vi "PCE_TCP_CMD.vi"(0 "CID IN":refnum<k5>, 7 "Timeout":u32=25 min=10 step=1, 11 "Error IN":errorcluster) -> (4 "CID OUT":refnum<k5>, 6 "FIFOelt":cluster{string, "data out":string, string}, 10 "Cmd?":bool, 15 "Error OUT":errorcluster)   [LabVIEW 2011]
panel:
  out "ExecTime":u32
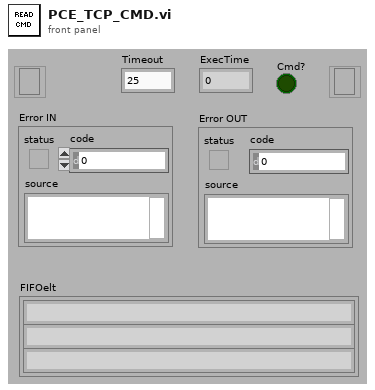
[diagram p1: front panel]
types:
  T1 = enum16{"Standard", "Buffered", "CRLF", "Immediate"}
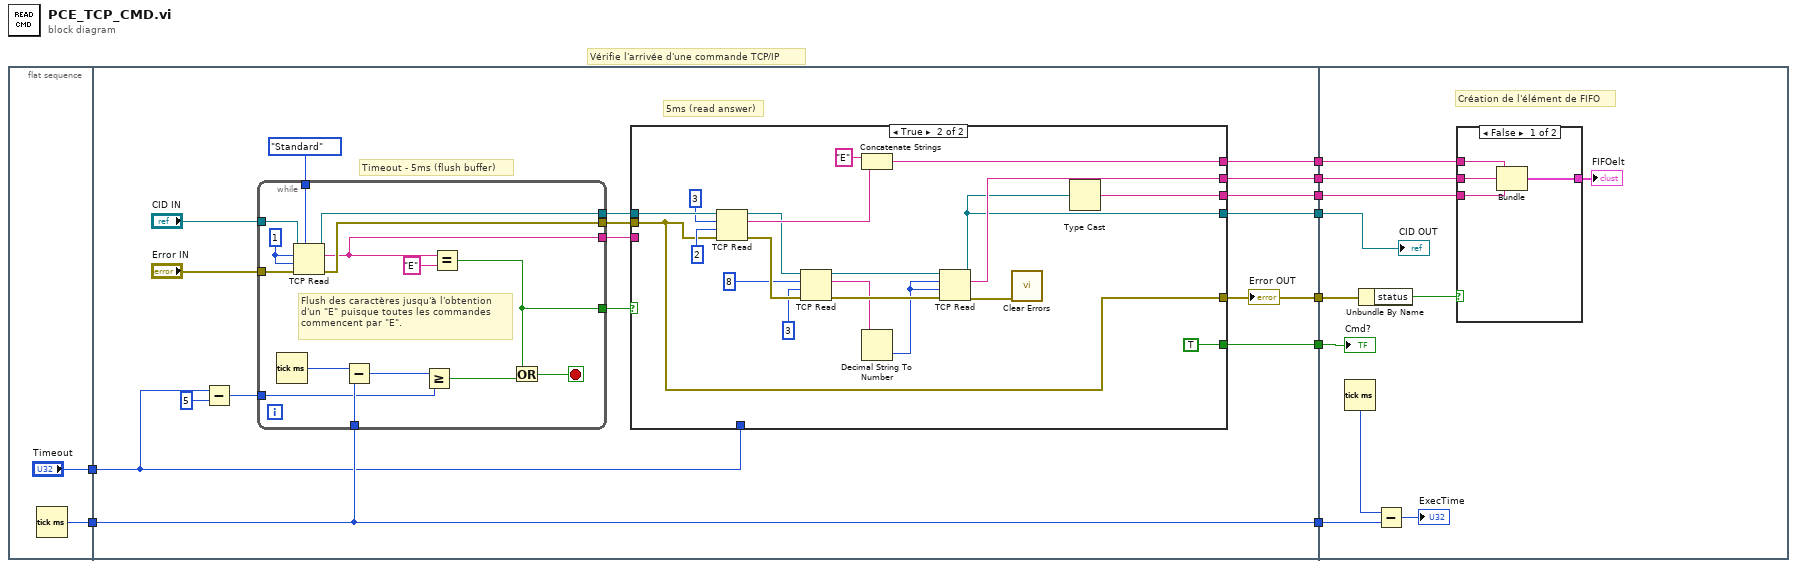
[diagram p0: block diagram]
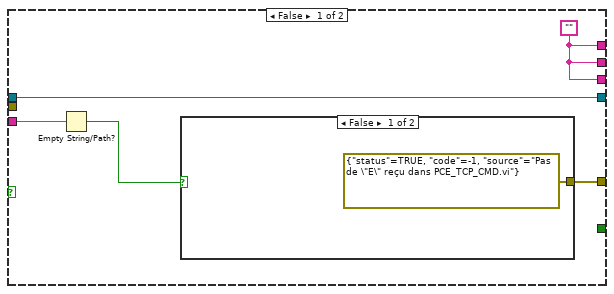
[diagram p2: hidden frame]
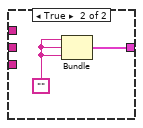
[diagram p4: hidden frame]
diagram:
  # "Vérifie l'arrivée d'une commande TCP/IP"
  n1 = flat-sequence {
    tunnel: [w11] -> w9
    tunnel: ["Timeout"] -> w7
    tunnel: w9 -> [w28]
    tunnel: [w28] -> w8
    tunnel: w7 -> [w20]
    tunnel: [w19] -> w6
    tunnel: [w18] -> w5
    tunnel: [w17] -> w4
    tunnel: [w16] -> w3
    tunnel: [w15] -> w2
    tunnel: [w12] -> w1
    tunnel: w8 -> [w80]
    tunnel: w6 -> [w71]
    tunnel: w5 -> [w77]
    tunnel: w4 -> [w75]
    tunnel: w3 -> [w74]
    tunnel: w2 -> [w73]
    tunnel: w1 -> [w70]
    frame #0 {
      n2 = Tick Count (ms)() -> (millisecond timer value=w11:u32)
    }
    frame #1 {
      # "5ms (read answer)"
      # "Timeout - 5ms (flush buffer)"
      n3 = Subtract(x=w20, y=u32 5) -> (x-y=w21:u32)
      n4 = while {
        tunnel: w28 -> [w42]
        tunnel: "CID IN" -> [w38]
        tunnel: T1."Standard" ("mode (standard)") -> [w37]
        tunnel: [w35] -> w25
        tunnel: [w34] -> w24
        tunnel: [w33] -> w23
        tunnel: w21 -> [w31]
        tunnel: "Error IN" -> [w30]
        tunnel: [w29] -> w13
        stop <- w40 stop-if-true
        w39 = 1 ("timeout ms (25000)")
        # "Flush des caractères jusqu'à l'obtention\nd'un \"E\" puisque toutes les commandes\ncommencent par \"E\"."
        n5 = Tick Count (ms)() -> (millisecond timer value=w43:u32)
        n6 = TCP Read(connection ID=w38, bytes to read=w39, error in (no error)=w30, 7:w37, 9:w39) -> (connection ID out=w34:refnum<k5>, data out=w29:string, error out=w33:errorcluster)
        n7 = Subtract(x=w43, y=w42) -> (x-y=w32:u32)
        n8 = Greater Or Equal?(x=w32, y=w31) -> (x >= y?=w41:bool)
        n9 = Equal?(x=w29, y="E") -> (x = y?=w35:bool)
        n10 = Or(x=w35, y=w41) -> (x .or. y?=w40:bool)
      }
      n11 = case shown="True" w25 {
        tunnel: w24 -> [w48 w69]
        tunnel: w23 -> [_ w51]
        tunnel: [w46 w51] -> w18
        tunnel: w20 -> [_ _]
        tunnel: [w48 w54] -> w19
        tunnel: [w47 w56] -> w17
        tunnel: [w47 w55] -> w16
        tunnel: [w47 w53] -> w15
        tunnel: w13 -> [w45 _]
        tunnel: [_ TRUE] -> w12
        frame False {
          w47 = ""
          n12 = Empty String/Path?(string/path=w45) -> (empty?=w44:bool)
          n13 = case shown="False" w44 {
            tunnel: [errorcluster {"status"=TRUE, "code"=-1, "source"="Pas de \"E\" reçu dans PCE_TCP_CMD.vi"} ("error out") _] -> w46
            frame False {
            }
            frame True {
            }
          }
        }
        frame True {
          n14 = TCP Read(connection ID=w69, bytes to read=3 ("length (rest)"), error in (no error)=w51, 9:2 ("timeout ms (25000)")) -> (connection ID out=w57:refnum<k5>, data out=w66:string, error out=w64:errorcluster)  [unwired: 1 in]
          n15 = TCP Read(connection ID=w57, bytes to read=8, error in (no error)=w64, 9:3 ("timeout ms (25000)")) -> (connection ID out=w61:refnum<k5>, data out=w59:string, error out=w60:errorcluster)  [unwired: 1 in]
          n16 = Concatenate Strings("E" ("string"), w66) -> (w56:string)
          n17 = Decimal String To Number(string=w59) -> (number=w58:i32)  [unwired: 2 in, 1 out]
          n18 = TCP Read(connection ID=w61, bytes to read=w58, error in (no error)=w60, 9:w58) -> (connection ID out=w54:refnum<k5>, data out=w55:string, error out=w50:errorcluster)  [unwired: 1 in]
          n19 = call <vilib>:"Clear Errors.vi"("error in (no error)"=w50) -> ()  [unwired: 6 in, 1 out]
          n20 = Type Cast(x=w54) -> (*(type *) &x=w53:string)  [unwired: 1 in]
        }
      }
      "Error OUT" <- w18
    }
    frame #2 {
      # "Création de l'élément de FIFO"
      n21 = Tick Count (ms)() -> (millisecond timer value=w79:u32)
      n22 = Unbundle By Name(w77) -> ("status"=w76:bool)
      n23 = Subtract(x=w79, y=w80) -> (x-y=→"ExecTime":u32)
      n24 = case shown="False" w76 {
        tunnel: w75 -> [w83 _]
        tunnel: w74 -> [w84 _]
        tunnel: w73 -> [w82 _]
        tunnel: [w81 w86] -> w72
        frame False {
          n25 = Bundle(w83, "data out"=w84, w82) -> (w81:cluster{string, "data out":string, string})  [unwired: 1 in]
        }
        frame True {
          w85 = ""
          n26 = Bundle(w85, w85, w85) -> (w86:cluster{string, string, string})  [unwired: 1 in]
        }
      }
      "FIFOelt" <- w72
      "CID OUT" <- w71
      "Cmd?" <- w70
    }
  }
